vi "State Selector.vi"(11 "Display State In":T1=enum."RPM") -> (2 "Changed?":bool, 3 "Display State Out":T1=enum."RPM")   [LabVIEW 2015]
doc: "This VI acts as a helper, taking in the previous display state and the state of DIO lines and returning the appropriate current display state. It also returns whether a new button has been pressed, which is used determine whether to update the display state in the RT VI."
uses:
  Custom Controls/Display State.ctl
  <vilib>/rvi/eio/common/nirviEmuTemplateMethod_errors.vi
  <vilib>/eio/EIONode/EIONode.xnode
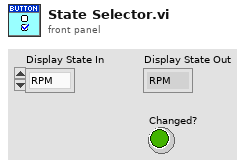
[diagram p1: front panel]
types:
  T1 = typedef "Display State.ctl" = enum16{"Battery State", "RPM", "Temp", "Voltage"}
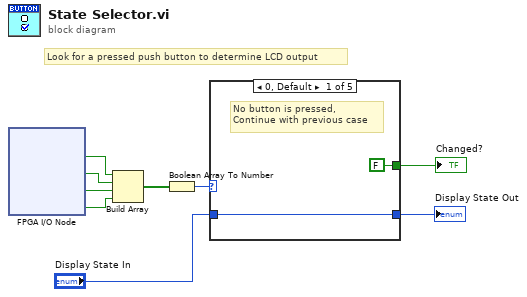
[diagram p0: block diagram]
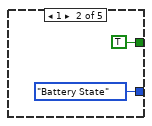
[diagram p2: hidden frame]
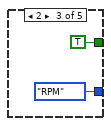
[diagram p3: hidden frame]
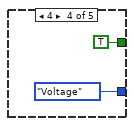
[diagram p4: hidden frame]
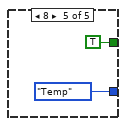
[diagram p5: hidden frame]
diagram:
  # "Look for a pressed push button to determine LCD output"
  n1 = xnode "FPGA I/O Node"() -> ("DIO12"=w7:bool, "DIO13"=w6:bool, "DIO15"=w8:bool, "DIO16"=w3:bool)  [unwired: 4 in, 4 out]
  n2 = Build Array(w7, w6, w8, w3) -> (w4:bool[])
  n3 = Boolean Array To Number(Boolean array=w4) -> (number=w9:u8)
  n4 = case shown="0, Default" w9 {
    tunnel: [w10 Display_State."Battery State" ("Display State In") Display_State."RPM" ("Display State In") Display_State."Voltage" ("Display State In") Display_State."Temp" ("Display State In")] -> w5
    tunnel: [FALSE TRUE TRUE TRUE TRUE] -> w2
    tunnel: "Display State In" -> [w10 _ _ _ _]
    frame 0, Default {
      # "No button is pressed, \nContinue with previous case"
    }
    frame 1 {
    }
    frame 2 {
    }
    frame 4 {
    }
    frame 8 {
    }
  }
  "Display State Out" <- w5
  "Changed?" <- w2
